vi "Read Rule parser.vi"(9 "Selection":string, 11 "UIManager in":refnum<class "UIManager.lvclass">) -> (0 "error out":errorcluster, 1 "Parameters":string, 2 "IRuleFileParser.lvclass":refnum<class "IRuleFileParser.lvclass">, 3 "UIManager out":refnum<class "UIManager.lvclass">, 4 "found?":bool)   [LabVIEW 2020, in "UserInterface.lvlib" / "UIManager.lvclass"]
uses:
  UIManager.lvclass
  ExtensionInterfaces/IRuleFileParser/IRuleFileParser.lvclass
  UIManager.lvclass/UIManager.ctl
  a68f1f4a-8182-4197-b8d3-3e0809a071fe.vi
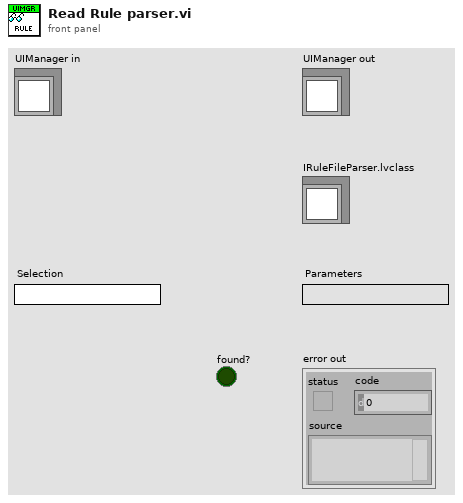
[diagram p1: front panel]
types:
  T1 = map{string, refnum<class "IRuleFileParser.lvclass">}
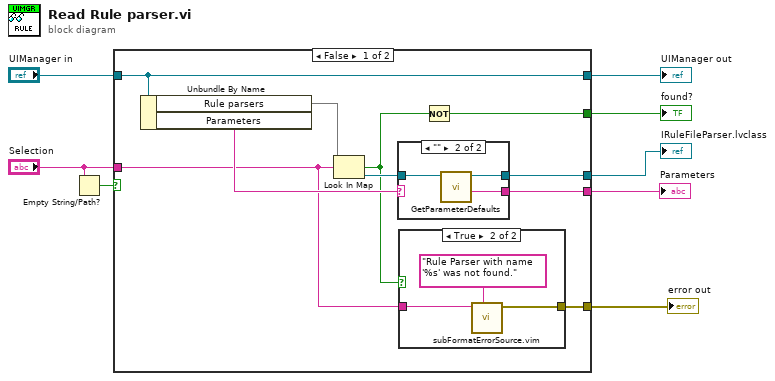
[diagram p0: block diagram]
diagram:
  n1 = Empty String/Path?(string/path="Selection") -> (empty?=w1:bool)
  n2 = case shown="False" w1 {
    tunnel: "UIManager in" -> [w9 w27]
    tunnel: [w17 _] -> w7
    tunnel: [w15 _] -> w6
    tunnel: [w13 _] -> w5
    tunnel: [w11 _] -> w4
    tunnel: "Selection" -> [w10 _]
    tunnel: [w9 w27] -> w3
    frame False {
      n3 = Unbundle By Name(w9) -> ("Rule parsers"=w18:T1, "Parameters"=w16:string)
      n4 = Look In Map(map=w18, key=w10) -> (key not found?=w12:bool, value=w14:refnum<class "IRuleFileParser.lvclass">)  [unwired: 1 in]
      n5 = case shown="\"\"" w16 {
        selector: w16 -> [w23 _]
        tunnel: [w23 w25] -> w15
        tunnel: w14 -> [w22 w26]
        tunnel: [w22 w24] -> w13
        frame Default {
        }
        frame "" {
          n6 = call-dynamic "GetParameterDefaults.vi"("IRuleFileParser in"=w26) -> ("Parameter defaults"=w25:string, "IRuleFileParser out"=w24:refnum<class "IRuleFileParser.lvclass">)  [unwired: 8 in, 1 out]
        }
      }
      n7 = case shown="True" w12 {
        tunnel: [_ w19] -> w11
        tunnel: w10 -> [_ w20]
        frame False {
        }
        frame True {
          n8 = call "subFormatErrorSource.vim"("format string"="Rule Parser with name '%s' was not found.", "Parameter cluster"=w20) -> ("Error out"=w19:errorcluster)  [unwired: 9 in]
        }
      }
      n9 = Not(x=w12) -> (.not. x?=w17:bool)
    }
    frame True {
    }
  }
  "UIManager out" <- w3
  "IRuleFileParser.lvclass" <- w5
  "found?" <- w7
  "Parameters" <- w6
  "error out" <- w4
